vi "带语音输入的命令整合.vi"(9 "CM":i32, 10 "step":i32, 11 "输入指令":string) -> (3 "命令":string)   [LabVIEW 2014]
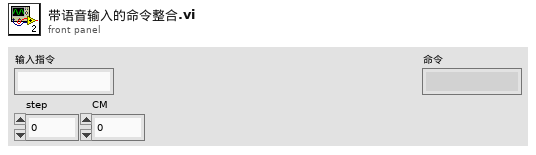
[diagram p1: front panel]
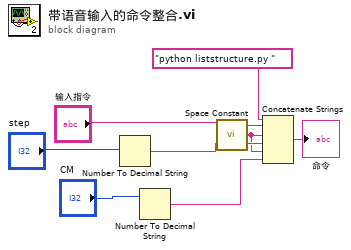
[diagram p0: block diagram]
diagram:
  n1 = Number To Decimal String(number="step") -> (decimal integer string=w7:string)  [unwired: 1 in]
  n2 = Number To Decimal String(number="CM") -> (decimal integer string=w5:string)  [unwired: 1 in]
  n3 = call <vilib>:"Space Constant.vi"() -> ("String"=w6:string)
  n4 = Concatenate Strings("python liststructure.py " ("command line"), "输入指令", w6, w7, w6, w5) -> (→"命令":string)
